vi "Tektronix 7000 Series Acquire Multiple Waveform.vi"() -> ()   [LabVIEW 2015]
doc: "Demonstrates how to set up an oscilloscope automatically. You can configure this VI to acquire multiple waveforms from several channels by following the following steps:\n\n1. Specify a valid VISA resource to use. \n2. Specify parameters in <B>Channel A</B>. \n3. Specify parameters in <B>Channel B</B>.\n4. Specify a time-out value for reading a waveform.\n5. Run this VI. The <B>Waveform Graph</B> displays the waveforms you acquire."
uses:
  <instrlib>/Tektronix 7000 Series/Public/Data/Read (Multiple Waveforms).vi
  <instrlib>/Tektronix 7000 Series/Tektronix 7000 Series.lvlib
panel:
  in  "Probe Attenuation (1.0) 2":dbl=1.0
  in  "Maximum Time (10000 ms)":u32=10000
  in  "Probe Attenuation (1.0)":dbl=1.0
  in  "Vertical Coupling (1: DC)":u16(ring)=1 items=["AC", "DC", "Ground"]
  in  "Vertical Coupling (1: DC)":u16(ring)=1 items=["AC", "DC", "Ground"]
  in  "Channel (1: Channel 2)":u16(ring)=1 items=["Channel 1", "Channel 2", "Channel 3", "Channel 4", "Math 1", "Math 2", "Math 3", "Math 4", "Reference 1", "Reference 2", "Reference 3", "Reference 4"]
  in  "Channel  (0: Channel 1)":u16(ring) items=["Channel 1", "Channel 2", "Channel 3", "Channel 4"]
  in  "VISA Resource Name":refnum<visa-resource-name>
  out "Waveform Graph":waveform(dbl)[](graph)
  # "(c) 2006. National Instruments Corporation. ALL RIGHTS RESERVED."
  # "(c) 2006 - 2016 National Instruments Corporation.  ALL RIGHTS RESERVED."
  # "Channel A"
  # "Channel B"
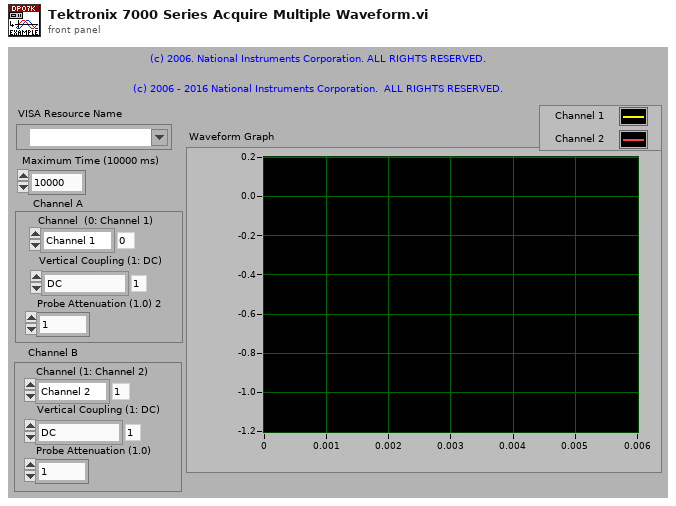
[diagram p1: front panel]
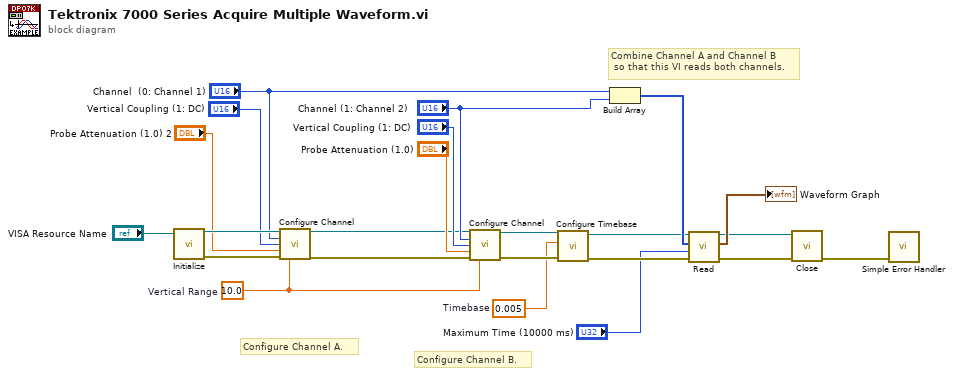
[diagram p0: block diagram]
diagram:
  w5 = 0.005  # Timebase
  w6 = 10.0  # Vertical Range
  # "Configure Channel A."
  # "Configure Channel B."
  # "Combine Channel A and Channel B\n so that this VI reads both channels."
  n1 = call <instrlib>:"Initialize.vi"("VISA resource name"="VISA Resource Name") -> ("error out"=w22:errorcluster, "VISA resource name out"=w21:refnum<visa-resource-name>)  [unwired: 9 in]
  n2 = call <instrlib>:"Configure Channel.vi"("VISA resource name"=w21, "Channel (0: Channel 1)"="Channel  (0: Channel 1)", "Vertical Coupling (1: DC)"="Vertical Coupling (1: DC)", "Probe Attenuation (1.0)"="Probe Attenuation (1.0) 2", "error in (no error)"=w22, "Vertical Range (10.0 V)"=w6) -> ("VISA resource name out"=w4:refnum<visa-resource-name>, "error out"=w3:errorcluster)  [unwired: 8 in]
  n3 = call <instrlib>:"Configure Channel.vi"("VISA resource name"=w4, "Channel (0: Channel 1)"="Channel (1: Channel 2)", "Vertical Coupling (1: DC)"="Vertical Coupling (1: DC)", "Probe Attenuation (1.0)"="Probe Attenuation (1.0)", "error in (no error)"=w3, "Vertical Range (10.0 V)"=w6) -> ("VISA resource name out"=w14:refnum<visa-resource-name>, "error out"=w13:errorcluster)  [unwired: 8 in]
  n4 = call <instrlib>:"Configure Timebase.vi"("error in (no error)"=w13, "Timebase (4 ns)"=w5, "VISA resource name"=w14) -> ("error out"=w11:errorcluster, "VISA resource name out"=w12:refnum<visa-resource-name>)  [unwired: 7 in]
  n5 = Build Array("Channel  (0: Channel 1)", "Channel (1: Channel 2)") -> (w20:u16[])
  n6 = call-poly <instrlib>:"Read.vi"("error in (no error)"=w11, "Maximum Time (10000 ms)"="Maximum Time (10000 ms)", "Channels"=w20, "VISA resource name"=w12) -> ("error out"=w17:errorcluster, "Waveform Data"=→"Waveform Graph":waveform(dbl)[], "VISA resource name out"=w18:refnum<visa-resource-name>)  [unwired: 5 in]
  n7 = call <instrlib>:"Close.vi"("error in (no error)"=w17, "VISA resource name"=w18) -> ("error out"=w16:errorcluster)  [unwired: 9 in]
  n8 = call <vilib>:"Simple Error Handler.vi"("error in (no error)"=w16) -> ()  [unwired: 4 in, 5 out]
